vi "shared-variable-host.vi"() -> ()   [LabVIEW 2015]
uses:
  controls/boolean_info.ctl
panel:
  out "booleen-errors":T1
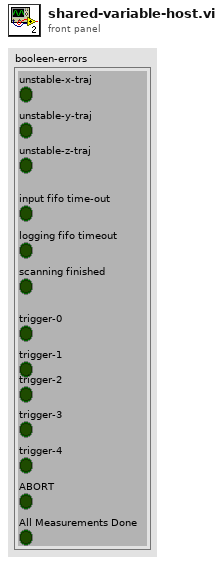
[diagram p1: front panel]
types:
  T1 = typedef "boolean_info.ctl" = cluster{"unstable-z-traj":bool, "input fifo time-out":bool, "logging fifo timeout":bool, "scanning finished":bool, "trigger-1":bool, "trigger-0":bool, "trigger-2":bool, "trigger-3":bool, "trigger-4":bool, "unstable-x-traj":bool, "unstable-y-traj":bool, "ABORT":bool, "All Measurements Done":bool}
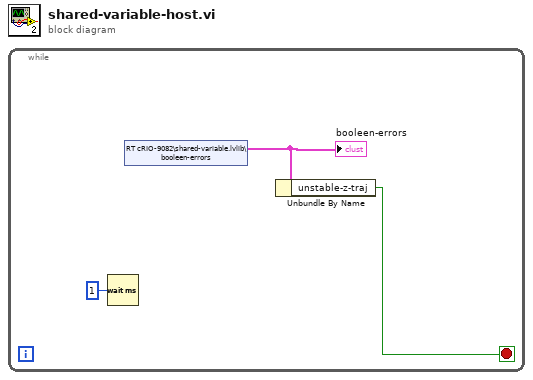
[diagram p0: block diagram]
diagram:
  n1 = while {
    stop <- w2 stop-if-true
    n2 = Wait (ms)(milliseconds to wait=u32 1) -> ()  [unwired: 1 out]
    n3 = shared-variable "RT cRIO-9082\\shared-variable.lvlib\\booleen-errors"() -> (w3:T1)  [unwired: 1 in, 1 out]
    "booleen-errors" <- w3
    n4 = Unbundle By Name(w3) -> ("unstable-z-traj"=w2:bool)
  }
